vi "Convert Time Cluster to Time String.vi"(8 "error in (no error)":errorcluster, 10 "Time":cluster{"Hour":i32, "Min":i32, "Sec":i32}, 11 "String":string) -> (0 "error out":errorcluster, 3 "Time String":string)   [LabVIEW 2020, in "Yokogawa GX Series.lvlib"]
doc: "Convert time cluster to string and concat after string."
uses:
  <instrlib>/Yokogawa GX Series/Yokogawa GX Series.lvlib
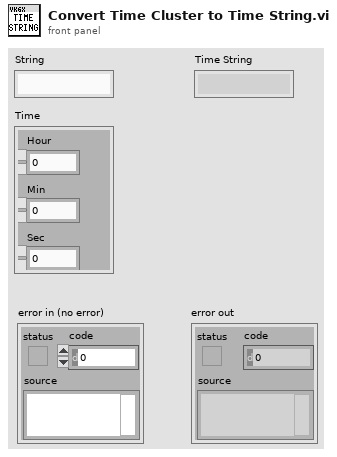
[diagram p1: front panel]
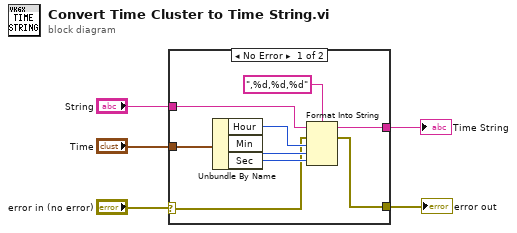
[diagram p0: block diagram]
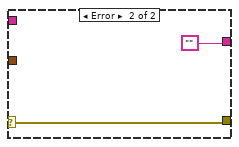
[diagram p2: hidden frame]
diagram:
  n1 = case shown="No Error" "error in (no error)" {
    selector: "error in (no error)" -> [w6 w16]
    tunnel: "Time" -> [w14 _]
    tunnel: [w10 w16] -> w4
    tunnel: [w9 ""] -> w3
    tunnel: "String" -> [w7 _]
    frame No Error {
      n2 = Unbundle By Name(w14) -> ("Hour"=w13:i32, "Min"=w12:i32, "Sec"=w11:i32)
      n3 = Format Into String(format string=",%d,%d,%d", initial string=w7, error in=w6, w13, w12, w11) -> (resulting string=w9:string, error out=w10:errorcluster)
    }
    frame Error {
    }
  }
  "Time String" <- w3
  "error out" <- w4
